vi "Create queue (SubVI).vi"(0 "Channel in":refnum<class "Channel.lvclass">, 1 "autoDelete (F)":bool, 2 "queue":string, 3 "error in (no error)":errorcluster, 4 "exclusive (F)":bool) -> (5 "Queue out":refnum<class "Queue.lvclass">, 6 "error out":errorcluster)   [LabVIEW 2016]
doc: "Create a queue with properties."
uses:
  <vilib>/Distrio/LabbitMQ/Channel/Channel.lvclass
  <vilib>/Distrio/LabbitMQ/Queue/Queue.lvclass
  <vilib>/Distrio/LabbitMQ/Channel/queue_declare_cluster.ctl
panel:
  in  "durable (F)":bool
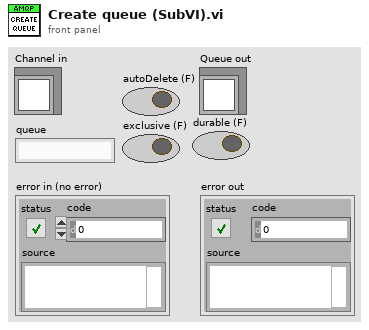
[diagram p1: front panel]
types:
  T1 = typedef "Channel.lvclass/queue_declare_cluster.ctl" = cluster{"queue":string, "durable (F)":bool, "exclusive (F)":bool, "autoDelete (F)":bool, "561934e089]], mscorlib, Version=0.0.0.0, Culture=neutral, PublicKeyToken=b77a5c561934e089\targuments":refnum<k24>}
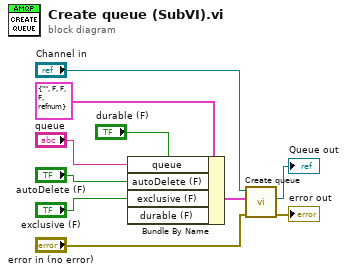
[diagram p0: block diagram]
diagram:
  n1 = Bundle By Name(cluster=T1 {"queue"="", "durable (F)"=FALSE, "exclusive (F)"=FALSE, "autoDelete (F)"=FALSE, "561934e089]], mscorlib, Version=0.0.0.0, Culture=neutral, PublicKeyToken=b77a5c561934e089\targuments"=refnum} ("QueueDeclare Properties"), "queue"="queue", "autoDelete (F)"="autoDelete (F)", "exclusive (F)"="exclusive (F)", "durable (F)"="durable (F)") -> (w5:T1)
  n2 = call <vilib>:"Create queue.vi"("error in (no error)"="error in (no error)", "QueueDeclare Properties"=w5, "Channel in"="Channel in") -> ("error out"=→"error out":errorcluster, "Queue.lvclass"=→"Queue out":refnum<class "Queue.lvclass">)  [unwired: 6 in, 1 out]
